vi "PPMS_ScanVoltage.vi"(6 "error in (no error)":errorcluster, 7 "Index":i8) -> (0 "error out":errorcluster, 1 "resulting string 2":string="                End scan volts", 2 "resulting string 1":string="                Scan Voltage from 0V to 1V at 0.5V/min, in 50 steps, Uniform", 3 "Cancelled?":bool)   [LabVIEW 2017]
doc: "Use this template to create a dialog box. This template polls the state of the buttons on the front panel and does not use events. Use the Dialog Using Events template (not available in Base package) to create a dialog box with event handling."
panel:
  in  "Modo de barrido":i32(ring) items=["Solo ir", "Ir y volver"]
  in  "Rate (V/min)":dbl=0.5
  in  "#puntos":u32=50
  in  "Voltaje Final (V)":dbl=1.0
  in  "Voltaje Inicial (V)":dbl
  in  "Cancel":bool
  in  "OK":bool
  # "Noviembre 2020 V1.3  a-sslcdms"
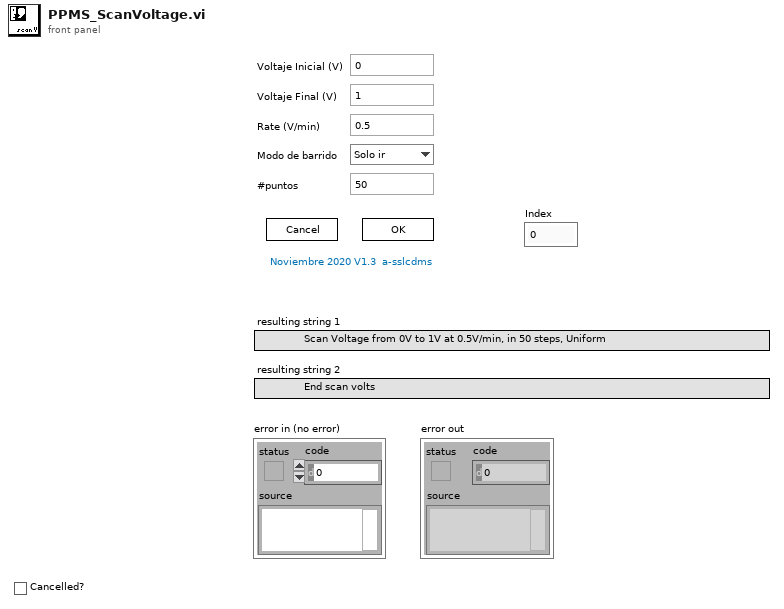
[diagram p1: front panel]
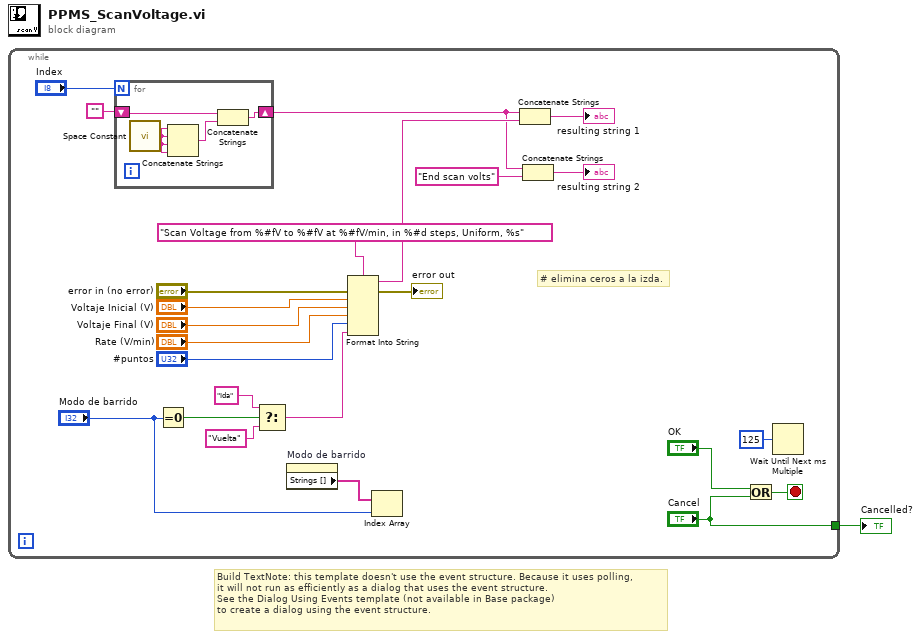
[diagram p0: block diagram]
diagram:
  # "Build TextNote: this template doesn't use the event structure. Because it uses polling, \nit will not run as efficiently as a dialog that uses the event structure.\nSee the Dialog Using Events template (not available in Base package) \nto create a dialog using the event structure."
  n1 = while {
    tunnel: ["Cancel"] -> w1
    stop <- w24 stop-if-true
    # "# elimina ceros a la izda."
    n2 = for {
      N: "Index" -> [_]
      shift-right: [w28] -> w12
      shift-left: "" -> [w27]
      n3 = call <vilib>:"Space Constant.vi"() -> ("String"=w26:string)
      n4 = Concatenate Strings(w26, w26, w26, w26) -> (w29:string)
      n5 = Concatenate Strings(w27, w29) -> (w28:string)
    }
    n6 = Equal To 0?(x="Modo de barrido") -> (x = 0?=w7:bool)
    n7 = Select(t="Ida" ("resulting string 2"), s=w7, f="Vuelta" ("resulting string 2")) -> (s? t:f=w2:string)
    n8 = property on="Modo de barrido" class="Ring (strict)"() -> ("Strings []"=w3:string[])  [unwired: 2 in, 2 out]
    n9 = Format Into String(format string="Scan Voltage from %#fV to %#fV at %#fV/min, in %#d steps, Uniform, %s", error in="error in (no error)", "Voltaje Inicial (V)", "Voltaje Final (V)", "Rate (V/min)", "#puntos", w2) -> (resulting string=w16:string, error out=→"error out":errorcluster)  [unwired: 1 in]
    n10 = Index Array(array=w3, index="Modo de barrido") -> ()  [unwired: 1 out]
    n11 = Concatenate Strings(w12, w16) -> (→"resulting string 1":string)
    n12 = Concatenate Strings(w12, "End scan volts" ("resulting string 2")) -> (→"resulting string 2":string)
    n13 = Or(x="OK", y="Cancel") -> (x .or. y?=w24:bool)
    n14 = Wait Until Next ms Multiple(millisecond multiple=u32 125) -> ()  [unwired: 1 out]
  }
  "Cancelled?" <- w1
